vi "Fix System Definition deployment issue.vi"(8 "error in (no error)":errorcluster, 11 "SysDef path in":path) -> (0 "error out":errorcluster, 3 "SysDef path out":path)   [LabVIEW 2019, in "Instrument Addon Specific System Tests.lvclass"]
uses:
  Instrument Addon Specific System Tests.lvclass
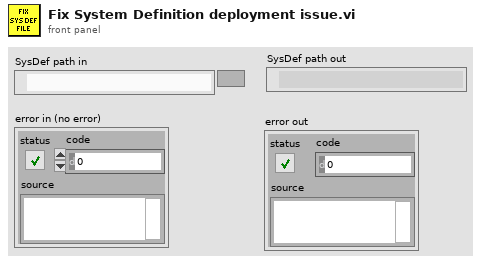
[diagram p1: front panel]
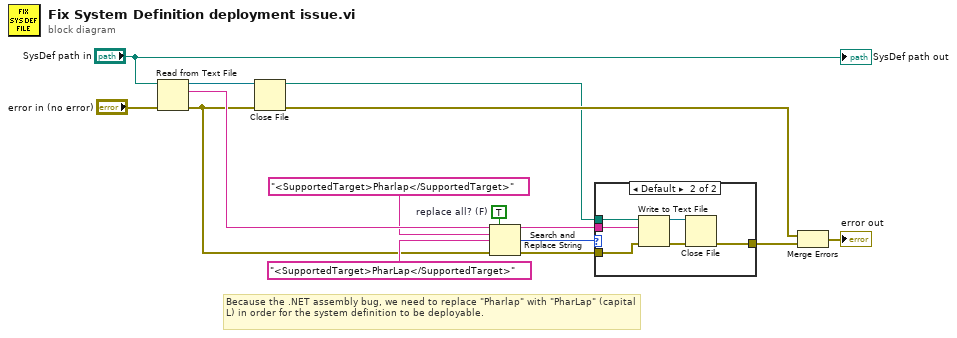
[diagram p0: block diagram]
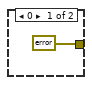
[diagram p2: hidden frame]
diagram:
  w13 = TRUE  # replace all? (F)
  # "Because the .NET assembly bug, we need to replace \"Pharlap\" with \"PharLap\" (capital L) in order for the system definition to be deployable."
  n1 = Read from Text File(file (use dialog)="SysDef path in", error in="error in (no error)") -> (refnum out=w15:refnum<file>, text=w10:string, error out=w6:errorcluster)  [unwired: 2 in, 1 out]
  n2 = Close File(refnum=w15, error in=w6) -> (path=w2:path, error out=w4:errorcluster)
  n3 = Search and Replace String(replace all?=w13, input string=w10, search string="<SupportedTarget>Pharlap</SupportedTarget>", replace string="<SupportedTarget>PharLap</SupportedTarget>" ("search string"), error in=w6) -> (result string=w12:string, number of replacements=w1:i32, error out=w11:errorcluster)  [unwired: 3 in, 1 out]
  n4 = case shown="Default" w1 {
    tunnel: w12 -> [_ w20]
    tunnel: w11 -> [_ w19]
    tunnel: [errorcluster {"status"=FALSE, "code"=0, "source"=""} ("error out") w18] -> w7
    tunnel: w2 -> [_ w17]
    frame 0 {
    }
    frame Default {
      n5 = Write to Text File(file (use dialog)=w17, text=w20, error in=w19) -> (refnum out=w21:refnum<file>, error out=w22:errorcluster)  [unwired: 1 in, 1 out]
      n6 = Close File(refnum=w21, error in=w22) -> (error out=w18:errorcluster)  [unwired: 1 out]
    }
  }
  n7 = Merge Errors(w4, w7) -> (→"error out":errorcluster)
  "SysDef path out" <- "SysDef path in"
